vi "启动界面.vi"() -> ()   [LabVIEW 2010]
panel:
  out "名称":string
  out "拆分的路径":path
  in  "密码":string
  in  "用户名":string
  in  "退出":bool
  in  "登录":bool
  # "登陆界面"
  # "用户名："
  # "密码："
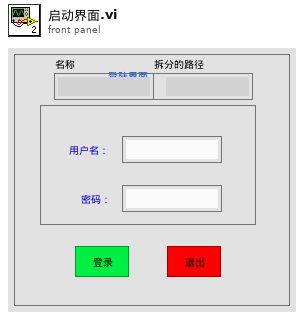
[diagram p1: front panel]
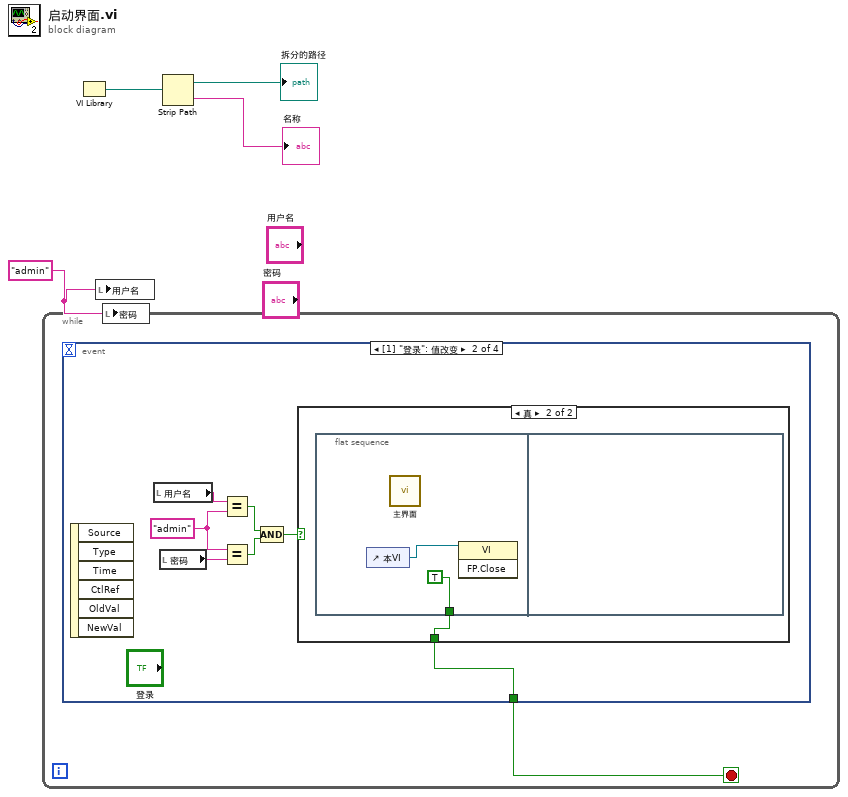
[diagram p0: block diagram]
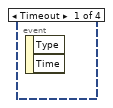
[diagram p2: hidden frame]
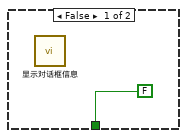
[diagram p3: hidden frame]
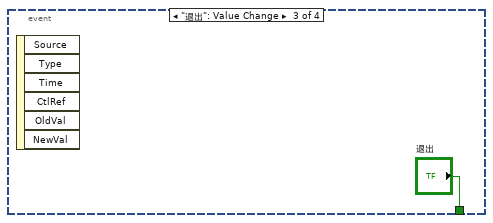
[diagram p4: hidden frame]
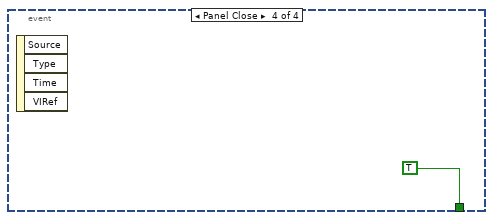
[diagram p5: hidden frame]
diagram:
  w4 = "admin"
  n1 = while {
    stop <- w5 stop-if-true
    n2 = event shown="[1] \"登录\": 值改变" {
      selector: _ -> [_ _ _ _]
      dyn-events: _ -> [_ _ _ _]
      timeout: _ -> [_ _ _ _]
      tunnel: [_ w6 "退出" TRUE] -> w5
      event Timeout {
        n3 = event-data() -> ()  [unwired: 1 in, 2 out]
      }
      event "登录": Value Change {
        w10 = "admin"
        n4 = event-data() -> ()  [unwired: 1 in, 6 out]
        n5 = local read "用户名"() -> (w12:string)
        n6 = local read "密码"() -> (w11:string)
        n7 = Equal?(x=w12, y=w10) -> (x = y?=w9:bool)
        n8 = Equal?(x=w10, y=w11) -> (x = y?=w8:bool)
        n9 = Compound Arithmetic op=AND(w9, w8) -> (w7:bool)
        n10 = case shown="真" w7 {
          tunnel: [FALSE w14] -> w6
          frame False {
            n11 = call "显示对话框信息"() -> ()  [unwired: 10 in, 2 out]
          }
          frame True {
            n12 = flat-sequence {
              tunnel: [TRUE] -> w14
              frame #0 {
                n13 = control-ref of="本VI"() -> (w15:refnum<vi>)
                n14 = call "主界面.vi"() -> ()  [unwired: 1 in]
                n15 = invoke class="VI" method="FP.Close"(reference=w15) -> ()  [unwired: 2 in, 3 out]
              }
              frame #1 {
              }
            }
          }
        }
      }
      event "退出": Value Change {
        n16 = event-data() -> ()  [unwired: 1 in, 6 out]
      }
      event Panel Close {
        n17 = event-data() -> ()  [unwired: 1 in, 4 out]
      }
    }
  }
  n18 = VI Library() -> (path=w3:path)
  n19 = local write "用户名"(w4) -> ()
  n20 = local write "密码"(w4) -> ()
  n21 = Strip Path(path=w3) -> (stripped path=→"拆分的路径":path, name=→"名称":string)
